vi "SingleMoleFinder.vi"(0 "Color Plane (IntensityExtraction)":i32(ring)=6 items=["Red", "Green", "Blue", "Hue", "Saturation", "Luminance", "Value", "Intensity"], 1 "Kernel (SmothingGaussian)":sgl[][](array[numeric])=[[1.0, 2.0, 4.0, 2.0, 1.0], [2.0, 4.0, 8.0, 4.0, 2.0], [4.0, 8.0, 16.0, 8.0, 4.0], [2.0, 4.0, 8.0, 4.0, 2.0], [1.0, 2.0, 4.0, 2.0, 1.0]], 2 "Divider (SmothingGaussian)":sgl, 3 "Kernel (Convolution)":sgl[][](array[numeric])=[[-1.0, -1.0, -1.0, -1.0, -1.0], [-1.0, -1.0, -1.0, -1.0, -1.0], [-1.0, -1.0, 30.0, -1.0, -1.0], [-1.0, -1.0, -1.0, -1.0, -1.0], [-1.0, -1.0, -1.0, -1.0, -1.0]], 4 "Divider (Convolution)":sgl, 5 "Method (AutoTresholdMomentClustering)":i32(ring)=3 items=["clustering", "entropy", "metric", "moments", "inter-class variance"], 6 "Look For (AutoTresholdMomentClustering)":u32(ring) items=["Bright Objects", "Dark Objects"], 7 "error in":errorcluster, 8 "Operator (LogarithmicSmoother)":T4(ring)=enum."Log", 9 "X Value (LogarithmicSmoother)":sgl=1.5, 10 "Operation (closeObjects)":T3(ring)=enum."PClose", 11 "Structuring Element (closeObjects)":i32[][](array[numeric])=[[0, 1, 1, 1, 0], [1, 1, 1, 1, 1], [1, 1, 1, 1, 1], [1, 1, 1, 1, 1], [0, 1, 1, 1, 0]], 12 "Square/Hexa (Square) (closeObjects)":bool, 13 "Connectivity 4/8 (8) (RemoveBorderObjects)":bool=TRUE, 14 "Square/Hexa (Square) (RemoveSmallObjects)":bool=TRUE, 15 "Connectivity 4/8 (8) (RemoveSmallObjects)":bool=TRUE, 16 "Low Pass/High Pass (Low) (RemoveSmallObjects)":bool, 17 "Connectivity 4/8 (8) (FillHoles)":bool=TRUE, 18 "Min Radius (CircleDetection)":sgl=15.0, 19 "Max Radius (CircleDetection)":sgl=50.0, 21 "Keep/Remove Particles (Particle Filter 1)":bool=TRUE, 22 "Connectivity 4/8 (8) (Particle Filter 1)":bool=TRUE, 23 "Selection Values (Particle Filter 1)":T2(array[cluster])=[{"Measurement Parameter"=1, "Range Lower Value"=0.0, "Range Upper Value"=0.0, "Range"=FALSE, "Measurement Type"=FALSE}, {"Measurement Parameter"=0, "Range Lower Value"=15.0, "Range Upper Value"=100.0, "Range"=FALSE, "Measurement Type"=FALSE}] {"Measurement Parameter" items=["Center of Mass X", "Center of Mass Y", "First Pixel X", "First Pixel Y", "Bounding Rect Left", "Bounding Rect Top", "Bounding Rect Right", "Bounding Rect Bottom", "Max Feret Diameter Start X", "Max Feret Diameter Start Y", "Max Feret Diameter End X", "Max Feret Diameter End Y", "Max Horiz. Segment Length Left", "Max Horiz. Segment Length Right", "Max Horiz. Segment Length Row", "-", "Bounding Rect Width", "Bounding Rect Height", "Bounding Rect Diagonal", "Perimeter", "Convex Hull Perimeter", "Holes' Perimeter", "Max Feret Diameter", "Equivalent Ellipse Major Axis", "Equivalent Ellipse Minor Axis", "Equivalent Ellipse Minor Axis (Feret)", "Equivalent Rect Long Side", "Equivalent Rect Short Side", "Equivalent Rect Diagonal", "Equivalent Rect Short Side (Feret)", "Average Horiz. Segment Length", "Average Vert. Segment Length", "Hydraulic Radius", "Waddel Disk Diameter", "-", "Area", "Holes' Area", "Particle & Holes' Area", "Convex Hull Area", "Image Area", "-", "Number of Holes", "Number of Horiz. Segments", "Number of Vert. Segments", "-", "Orientation", "Max Feret Diameter Orientation", "-", "% Area/Image Area", "% Area/(Particle & Holes' Area)", "Ratio of Equivalent Ellipse Axes", "Ratio of Equivalent Rect Sides", "-", "Elongation Factor", "Compactness Factor", "Heywood Circularity Factor", "Type Factor", "-", "Sum X", "Sum Y", "Sum XX", "Sum XY", "Sum YY", "Sum XXX", "Sum XXY", "Sum XYY", "Sum YYY", "-", "Moment of Inertia XX", "Moment of Inertia XY", "Moment of Inertia YY", "Moment of Inertia XXX", "Moment of Inertia XXY", "Moment of Inertia XYY", "Moment of Inertia YYY", "Norm. Moment of Inertia XX", "Norm. Moment of Inertia XY", "Norm. Moment of Inertia YY", "Norm. Moment of Inertia XXX", "Norm. Moment of Inertia XXY", "Norm. Moment of Inertia XYY", "Norm. Moment of Inertia YYY", "Hu Moment 1", "Hu Moment 2", "Hu Moment 3", "Hu Moment 4", "Hu Moment 5", "Hu Moment 6", "Hu Moment 7"]}, 24 "Connectivity 4/8 (8) (ParticleTable)":bool=TRUE, 25 "Pixel Measurements (ParticleTable)":i32[](array[ring])=[0, 1, 2, 3, 4, 5, 6, 7, 8, 9, 10, 11, 12, 13, 14, 16, 17, 18, 19, 20, 21, 22, 23, 24, 25, 26, 27, 28, 29, 30, 31, 32, 33, 35, 36, 37, 38, 39, 41, 42, 43, 45, 46, 48, 49, 50, 51, 53, 54, 55, 56, 58, 59, 60, 61, 62, 63, 64, 65, 66, 68, 69, 70, 71, 72, 73, 74, 75, 76, 77, 78, 79, 80, 81, 82, 83, 84, 85, 86, 87, 88] items=["Center of Mass X", "Center of Mass Y", "First Pixel X", "First Pixel Y", "Bounding Rect Left", "Bounding Rect Top", "Bounding Rect Right", "Bounding Rect Bottom", "Max Feret Diameter Start X", "Max Feret Diameter Start Y", "Max Feret Diameter End X", "Max Feret Diameter End Y", "Max Horiz. Segment Length Left", "Max Horiz. Segment Length Right", "Max Horiz. Segment Length Row", "-", "Bounding Rect Width", "Bounding Rect Height", "Bounding Rect Diagonal", "Perimeter", "Convex Hull Perimeter", "Holes' Perimeter", "Max Feret Diameter", "Equivalent Ellipse Major Axis", "Equivalent Ellipse Minor Axis", "Equivalent Ellipse Minor Axis (Feret)", "Equivalent Rect Long Side", "Equivalent Rect Short Side", "Equivalent Rect Diagonal", "Equivalent Rect Short Side (Feret)", "Average Horiz. Segment Length", "Average Vert. Segment Length", "Hydraulic Radius", "Waddel Disk Diameter", "-", "Area", "Holes' Area", "Particle & Holes' Area", "Convex Hull Area", "Image Area", "-", "Number of Holes", "Number of Horiz. Segments", "Number of Vert. Segments", "-", "Orientation", "Max Feret Diameter Orientation", "-", "% Area/Image Area", "% Area/(Particle & Holes' Area)", "Ratio of Equivalent Ellipse Axes", "Ratio of Equivalent Rect Sides", "-", "Elongation Factor", "Compactness Factor", "Heywood Circularity Factor", "Type Factor", "-", "Sum X", "Sum Y", "Sum XX", "Sum XY", "Sum YY", "Sum XXX", "Sum XXY", "Sum XYY", "Sum YYY", "-", "Moment of Inertia XX", "Moment of Inertia XY", "Moment of Inertia YY", "Moment of Inertia XXX", "Moment of Inertia XXY", "Moment of Inertia XYY", "Moment of Inertia YYY", "Norm. Moment of Inertia XX", "Norm. Moment of Inertia XY", "Norm. Moment of Inertia YY", "Norm. Moment of Inertia XXX", "Norm. Moment of Inertia XXY", "Norm. Moment of Inertia XYY", "Norm. Moment of Inertia YYY", "Hu Moment 1", "Hu Moment 2", "Hu Moment 3", "Hu Moment 4", "Hu Moment 5", "Hu Moment 6", "Hu Moment 7"]) -> (20 "Nb Circles (CircleDetection)":i32, 26 "Circles Data (CircleDetection)":T1(array[cluster]), 27 "error out":errorcluster)   [LabVIEW 2013]
uses:
  <vilib>/vision/NI_Vision_Development_Module.lvlib
panel:
  out "Circles Data (calibrated)":T1(array[cluster])
  out "Number of Particles 2":i32
  out "Number of Particles":i32
  out "Particle Measurements (Pixels)":dbl[][](array[numeric]) format="%.2f"
  out "Particle Measurements (Real-World)":dbl[][](array[numeric]) format="%.2f"
  out "Image Out":T5(plugin-control)
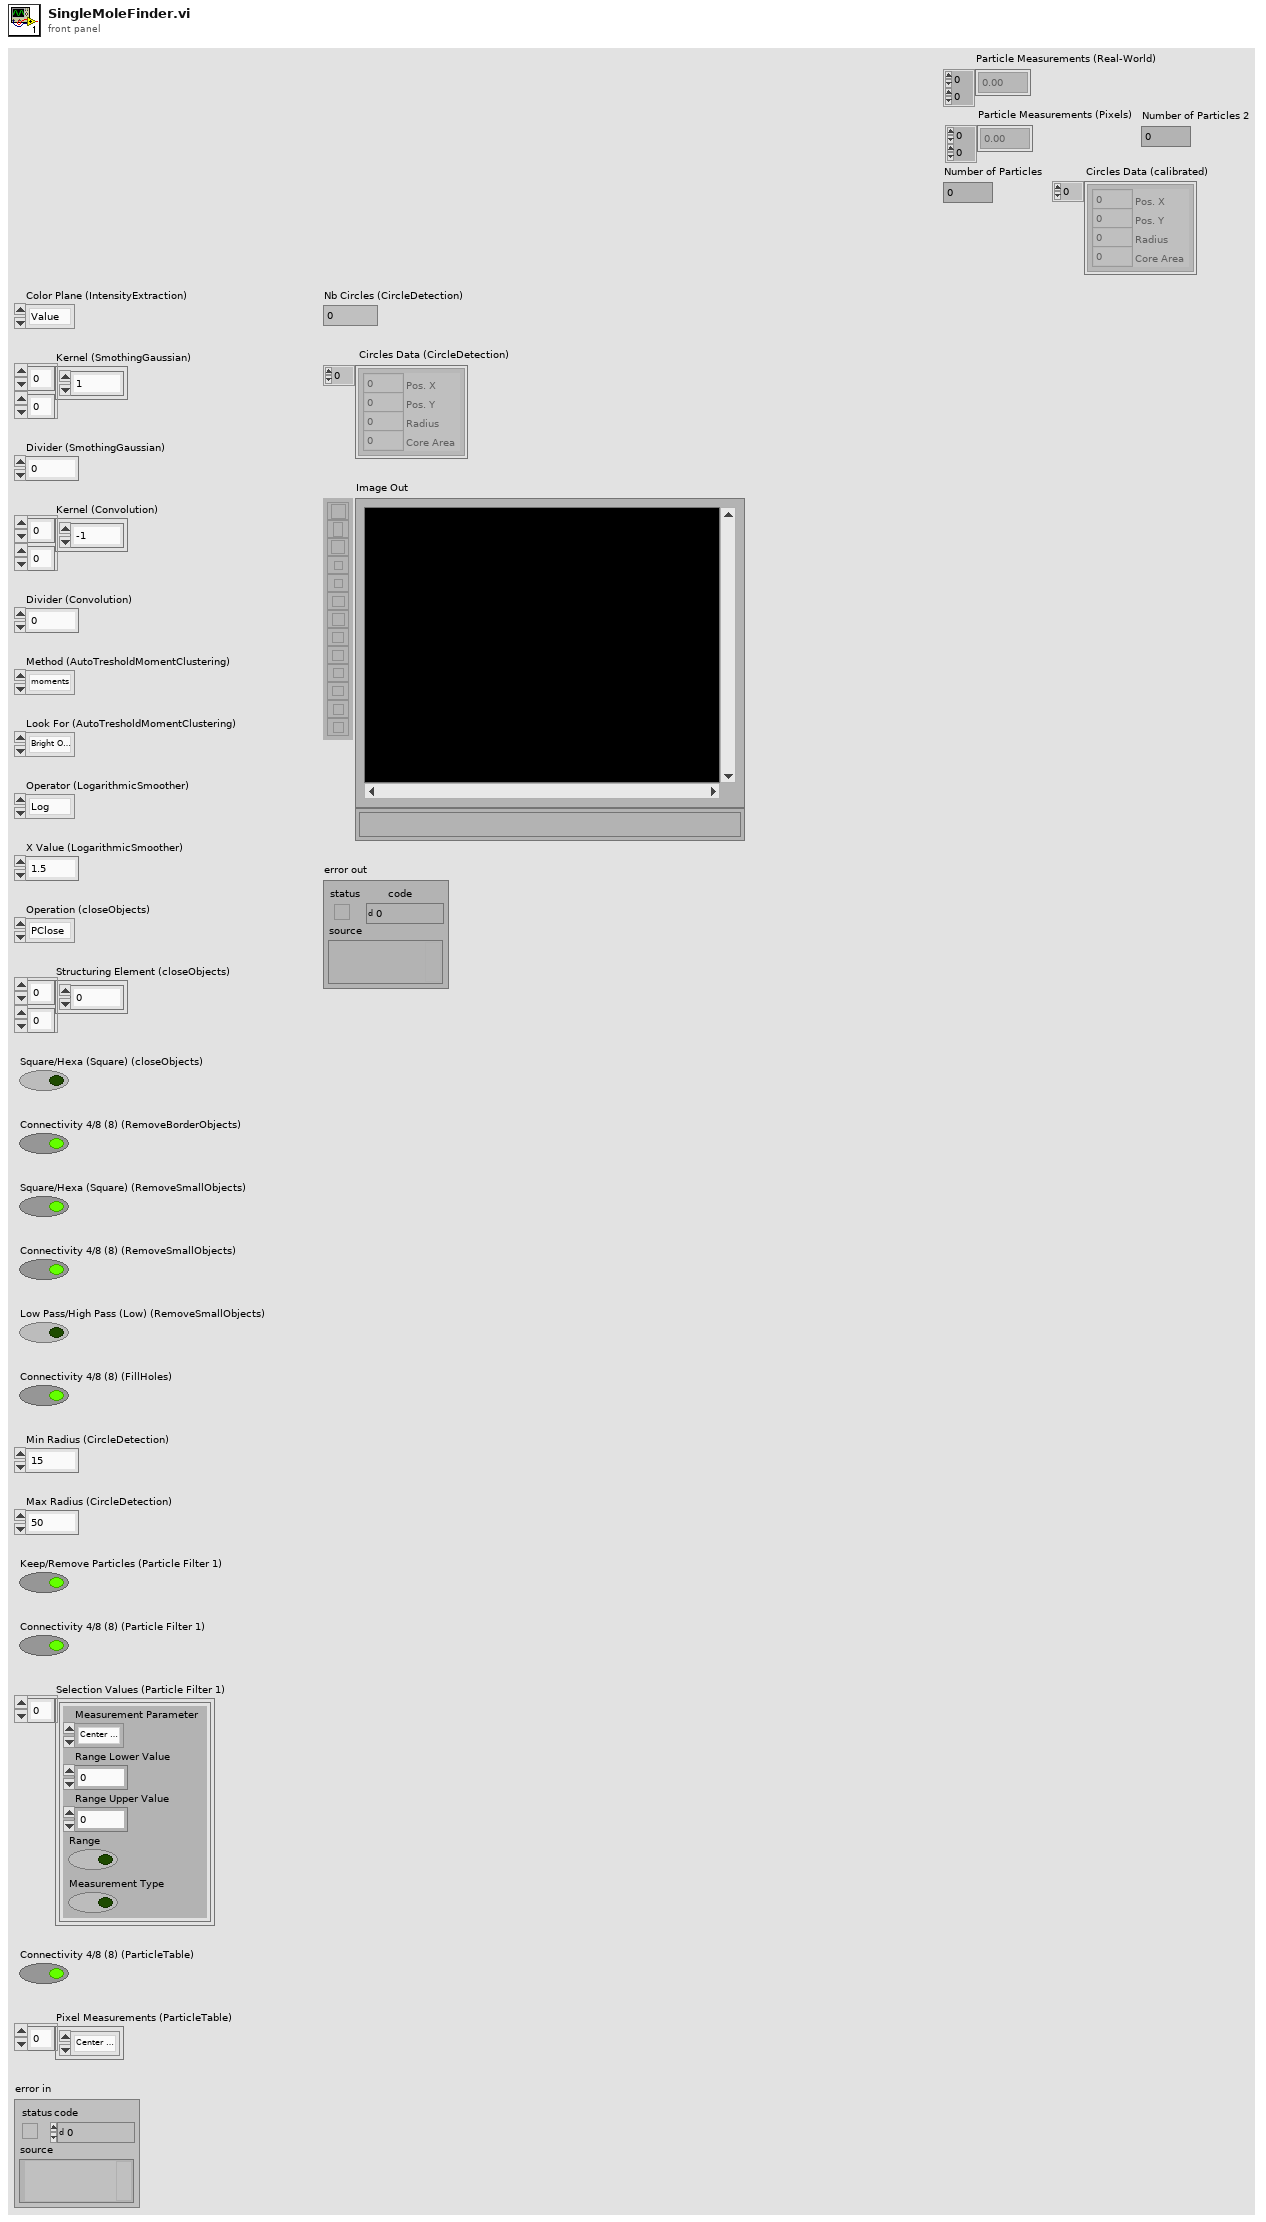
[diagram p1: front panel]
types:
  T1 = cluster{"Pos. X":i32, "Pos. Y":i32, "Radius":i32, "Core Area":i32}[]
  T2 = cluster{"Measurement Parameter":i32, "Range Lower Value":dbl, "Range Upper Value":dbl, "Range":bool, "Measurement Type":bool}[]
  T3 = enum32{"AutoM", "Close", "Dilate", "Erode", "Gradient", "Gradient out", "Gradient in", "Hit miss", "Open", "PClose", "POpen", "Thick", "Thin"}
  T4 = enum32{"Linear", "Log", "Exp", "Square", "Square root", "Power X", "Power 1/X"}
  T5 = typedef "IMAQ Image.ctl" = refnum<image>
  T6 = typedef "Image Type" = u32
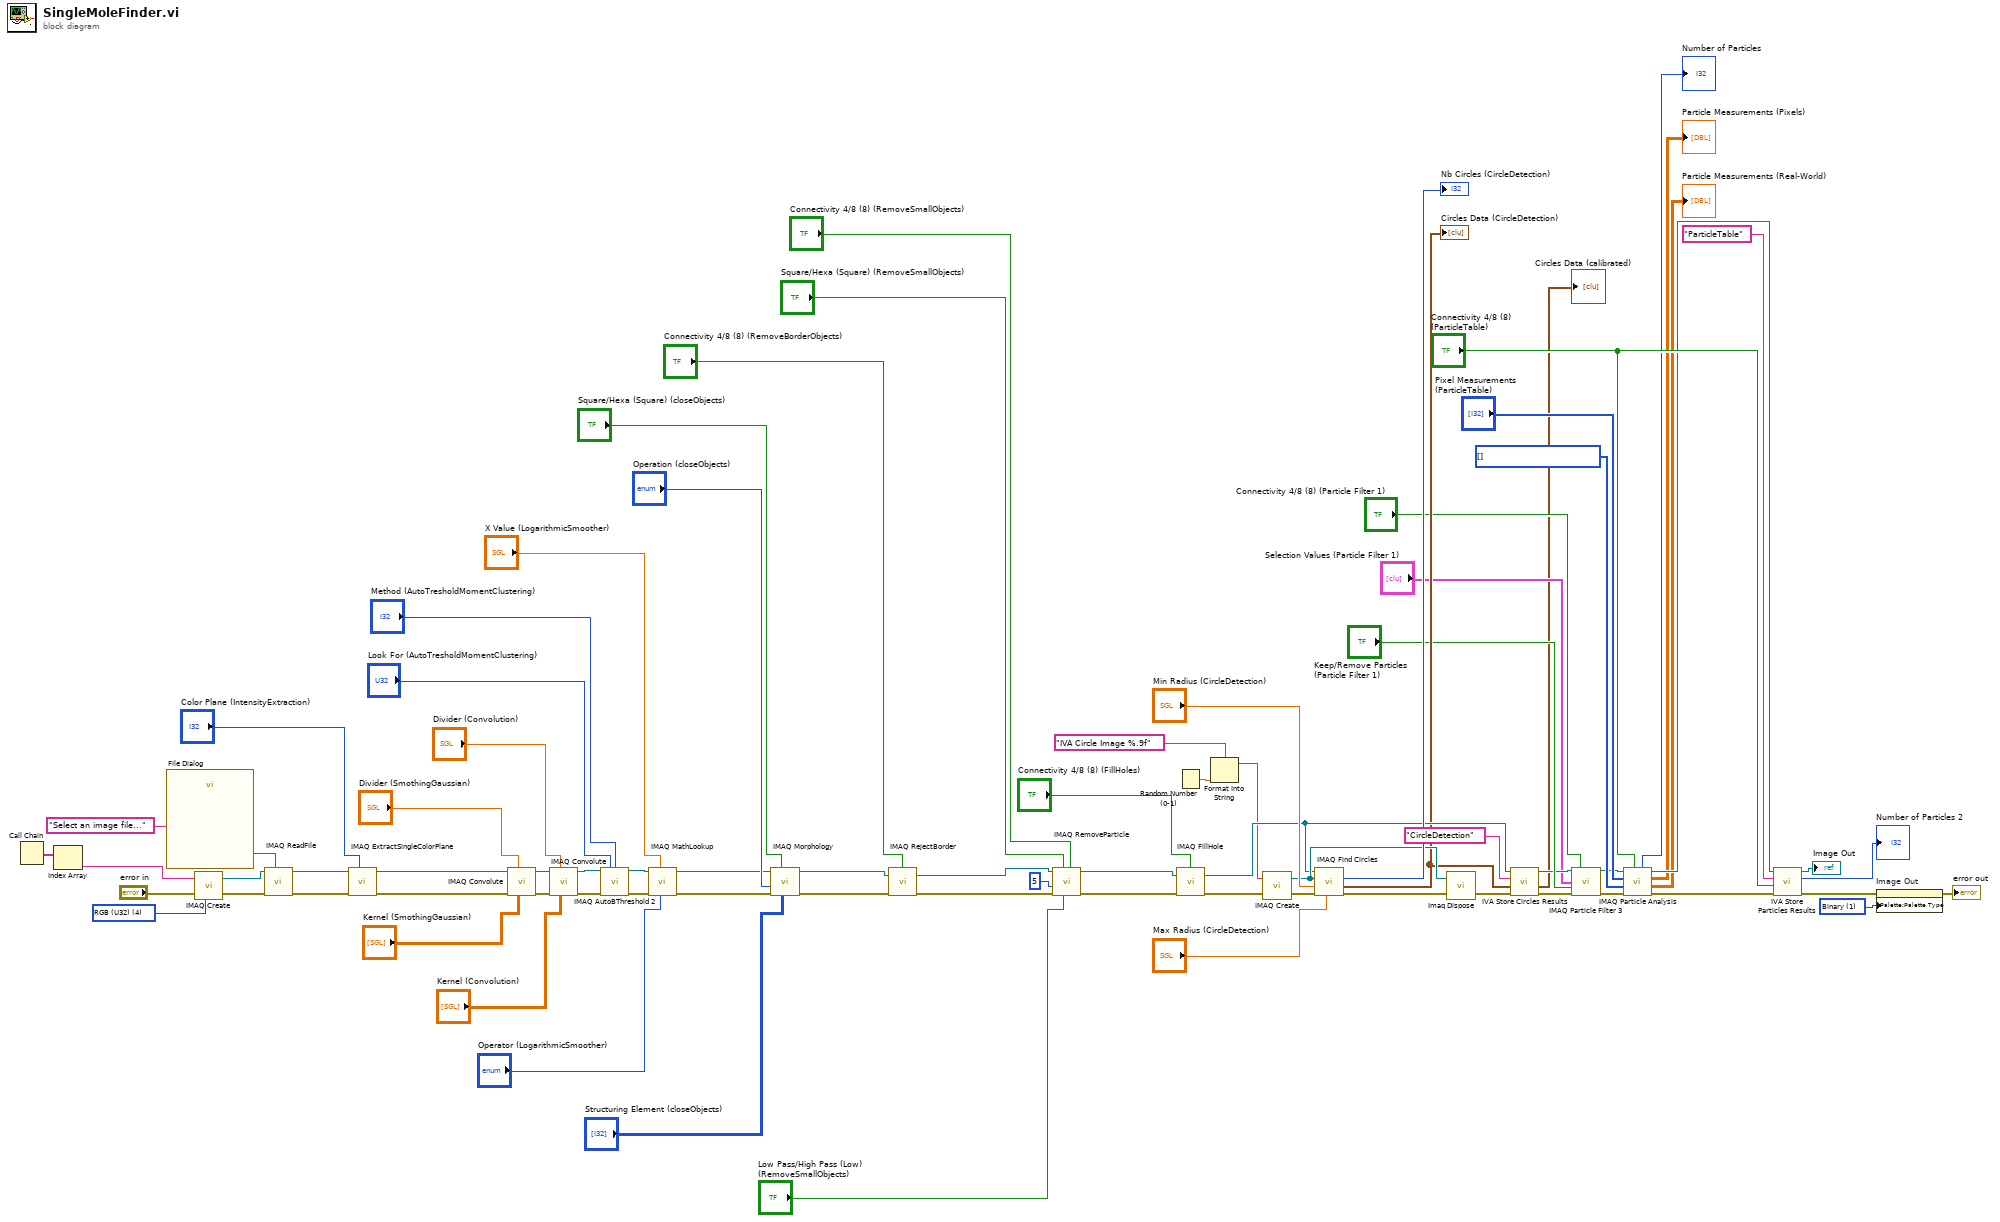
[diagram p0: block diagram]
diagram:
  w8 = u32 1 items=["Grayscale", "Binary", "Gradient", "Rainbow", "Temperature", "User Defined"] ("Palette")
  w16 = i32[] [] items=["Center of Mass X", "Center of Mass Y", "First Pixel X", "First Pixel Y", "Bounding Rect Left", "Bounding Rect Top", "Bounding Rect Right", "Bounding Rect Bottom", "Max Feret Diameter Start X", "Max Feret Diameter Start Y", "Max Feret Diameter End X", "Max Feret Diameter End Y", "Max Horiz. Segment Length Left", "Max Horiz. Segment Length Right", "Max Horiz. Segment Length Row", "-", "Bounding Rect Width", "Bounding Rect Height", "Bounding Rect Diagonal", "Perimeter", "Convex Hull Perimeter", "Holes' Perimeter", "Max Feret Diameter", "Equivalent Ellipse Major Axis", "Equivalent Ellipse Minor Axis", "Equivalent Ellipse Minor Axis (Feret)", "Equivalent Rect Long Side", "Equivalent Rect Short Side", "Equivalent Rect Diagonal", "Equivalent Rect Short Side (Feret)", "Average Horiz. Segment Length", "Average Vert. Segment Length", "Hydraulic Radius", "Waddel Disk Diameter", "-", "Area", "Holes' Area", "Particle & Holes' Area", "Convex Hull Area", "Image Area", "-", "Number of Holes", "Number of Horiz. Segments", "Number of Vert. Segments", "-", "Orientation", "Max Feret Diameter Orientation", "-", "% Area/Image Area", "% Area/(Particle & Holes' Area)", "Ratio of Equivalent Ellipse Axes", "Ratio of Equivalent Rect Sides", "-", "Elongation Factor", "Compactness Factor", "Heywood Circularity Factor", "Type Factor", "-", "Sum X", "Sum Y", "Sum XX", "Sum XY", "Sum YY", "Sum XXX", "Sum XXY", "Sum XYY", "Sum YYY", "-", "Moment of Inertia XX", "Moment of Inertia XY", "Moment of Inertia YY", "Moment of Inertia XXX", "Moment of Inertia XXY", "Moment of Inertia XYY", "Moment of Inertia YYY", "Norm. Moment of Inertia XX", "Norm. Moment of Inertia XY", "Norm. Moment of Inertia YY", "Norm. Moment of Inertia XXX", "Norm. Moment of Inertia XXY", "Norm. Moment of Inertia XYY", "Norm. Moment of Inertia YYY", "Hu Moment 1", "Hu Moment 2", "Hu Moment 3", "Hu Moment 4", "Hu Moment 5", "Hu Moment 6", "Hu Moment 7"] ("Real-World Measurements")
  w73 = T6 4 items=["Grayscale (U8)", "Grayscale (I16)", "Grayscale (SGL)", "Complex (CSG)", "RGB (U32)", "HSL (U32)", "RGB (U64)", "Grayscale (U16)"] ("Image Type")
  n1 = Call Chain() -> (call chain=w77:string[])
  n2 = Index Array(array=w77) -> (element=w76:string)  [unwired: 1 in]
  n3 = call "File Dialog"("prompt"="Select an image file...") -> ("selected path"=w74:path)  [unwired: 6 in, 8 out]
  n4 = call "IMAQ Create"("Image Name"=w76, "Image Type"=w73, "error in (no error)"="error in") -> ("New Image"=w80:T5, "error out"=w79:errorcluster)  [unwired: 1 in, 1 out]
  n5 = call "IMAQ ReadFile"("File Path"=w74, "error in (no error)"=w79, "Image"=w80) -> ("error out"=w70:errorcluster, "Image Out"=w71:T5)  [unwired: 2 in, 5 out]
  n6 = call "IMAQ ExtractSingleColorPlane"("Color Plane"="Color Plane (IntensityExtraction)", "error in (no error)"=w70, "Image Src"=w71) -> ("error out"=w67:errorcluster, "Image Dst Out"=w68:T5)  [unwired: 1 in, 6 out]
  n7 = call "IMAQ Convolute"("Kernel"="Kernel (SmothingGaussian)", "Divider (kernel sum)"="Divider (SmothingGaussian)", "error in (no error)"=w67, "Image Src"=w68) -> ("error out"=w63:errorcluster, "Image Dst Out"=w64:T5)  [unwired: 3 in, 3 out]
  n8 = call "IMAQ Convolute"("Kernel"="Kernel (Convolution)", "Divider (kernel sum)"="Divider (Convolution)", "error in (no error)"=w63, "Image Src"=w64) -> ("error out"=w61:errorcluster, "Image Dst Out"=w60:T5)  [unwired: 3 in, 3 out]
  n9 = call "IMAQ AutoBThreshold 2"("Image Src"=w60, "Look For (Bright Objects)"="Look For (AutoTresholdMomentClustering)", "Method (clustering)"="Method (AutoTresholdMomentClustering)", "error in (no error)"=w61) -> ("Image Dst Out"=w55:T5, "error out"=w54:errorcluster)  [unwired: 4 in, 6 out]
  n10 = call "IMAQ MathLookup"("Operator"="Operator (LogarithmicSmoother)", "X Value"="X Value (LogarithmicSmoother)", "error in (no error)"=w54, "Image Src"=w55) -> ("error out"=w49:errorcluster, "Image Dst Out"=w50:T5)  [unwired: 3 in, 3 out]
  n11 = call "IMAQ Morphology"("Structuring Element"="Structuring Element (closeObjects)", "Square/Hexa (Square)"="Square/Hexa (Square) (closeObjects)", "error in (no error)"=w49, "Operation"="Operation (closeObjects)", "Image Src"=w50) -> ("error out"=w46:errorcluster, "Image Dst Out"=w47:T5)  [unwired: 2 in, 3 out]
  n12 = call "IMAQ RejectBorder"("error in (no error)"=w46, "Image Src"=w47, "Connectivity 4/8 (8)"="Connectivity 4/8 (8) (RemoveBorderObjects)") -> ("error out"=w40:errorcluster, "Image Dst Out"=w41:T5)  [unwired: 1 in, 2 out]
  n13 = call "IMAQ RemoveParticle"("Connectivity 4/8 (8)"="Connectivity 4/8 (8) (RemoveSmallObjects)", "Low Pass/High Pass (Low)"="Low Pass/High Pass (Low) (RemoveSmallObjects)", "Square/Hexa (Square)"="Square/Hexa (Square) (RemoveSmallObjects)", "error in (no error)"=w40, "Number of Erosion"=5, "Image Src"=w41) -> ("error out"=w37:errorcluster, "Image Dst Out"=w38:T5)  [unwired: 1 in, 3 out]
  n14 = Random Number (0-1)() -> (number: 0 to 1=w23:dbl)
  n15 = call "IMAQ FillHole"("error in (no error)"=w37, "Image Src"=w38, "Connectivity 4/8 (8)"="Connectivity 4/8 (8) (FillHoles)") -> ("error out"=w31:errorcluster, "Image Dst Out"=w28:T5)  [unwired: 1 in, 2 out]
  n16 = Format Into String(format string="IVA Circle Image %.9f" ("Image Name"), w23) -> (resulting string=w25:string)  [unwired: 2 in, 1 out]
  n17 = call "IMAQ Create"("Image Name"=w25, "error in (no error)"=w31) -> ("New Image"=w33:T5, "error out"=w32:errorcluster)  [unwired: 2 in, 1 out]
  n18 = call "IMAQ Find Circles"("Max Radius"="Max Radius (CircleDetection)", "error in (no error)"=w32, "Min Radius"="Min Radius (CircleDetection)", "Image Dst"=w33, "Image Src"=w28) -> ("error out"=w30:errorcluster, "Circles Data"=w26:T1, "Nb Circles"=→"Nb Circles (CircleDetection)":i32)  [unwired: 4 out]
  "Circles Data (CircleDetection)" <- w26
  n19 = call "Imaq Dispose"("Image"=w33, "error in (no error)"=w30) -> ("error out"=w29:errorcluster)  [unwired: 1 in, 3 out]
  n20 = call <vilib>:"IVA Store Circles Results.vi"("error in (no error)"=w29, "Circles Data"=w26, "Step Name"="CircleDetection", "Image in"=w28) -> ("error out"=w19:errorcluster, "Circles Data (calibrated)"=→"Circles Data (calibrated)":T1, "Image dup"=w20:T5)  [unwired: 5 out]
  n21 = call "IMAQ Particle Filter 3"("Image Src"=w20, "Connectivity 4/8 (8)"="Connectivity 4/8 (8) (Particle Filter 1)", "Selection Values"="Selection Values (Particle Filter 1)", "Keep/Remove Particles (F)"="Keep/Remove Particles (Particle Filter 1)", "error in (no error)"=w19) -> ("Image Dst Out"=w14:T5, "error out"=w15:errorcluster)  [unwired: 4 in, 5 out]
  n22 = call "IMAQ Particle Analysis"("Connectivity 4/8 (8)"="Connectivity 4/8 (8) (ParticleTable)", "error in (no error)"=w15, "Real-World Measurements"=w16, "Pixel Measurements"="Pixel Measurements (ParticleTable)", "Image"=w14) -> ("error out"=w10:errorcluster, "Particle Measurements (Real-World)"=→"Particle Measurements (Real-World)":dbl[][], "Particle Measurements (Pixels)"=→"Particle Measurements (Pixels)":dbl[][], "Image Out (duplicate)"=w12:T5, "Number of Particles"=→"Number of Particles":i32)  [unwired: 2 out]
  n23 = call <vilib>:"IVA Store Particles Results.vi"("error in (no error)"=w10, "Connectivity 4/8 (8)"="Connectivity 4/8 (8) (ParticleTable)", "Step Name"="ParticleTable", "Image in"=w12) -> ("error out"=w7:errorcluster, "Number of Particles"=→"Number of Particles 2":i32, "Image dup"=→"Image Out":T5)  [unwired: 5 out]
  n24 = property on="Image Out" class="ImageControl"(error in=w7, "Palette:Palette Type"=w8) -> (error out=→"error out":errorcluster)  [unwired: 1 in, 1 out]
